vi "Event Receive.vi"(11 "Base Event jettl in":refnum<class "Base Event jettl.lvclass">) -> (2 "Event Msg Strategy":refnum<user-event>, 3 "Base Event jettl out":refnum<class "Base Event jettl.lvclass">)   [LabVIEW 2021, in "jettl.lvlib" / "Base Event jettl.lvlib" / "Base Event jettl.lvclass"]
uses:
  Base Event jettl.lvclass
  Msg Strategy/Msg Strategy/Msg Strategy.lvclass
  Base Event jettl.lvclass/Base Event jettl.ctl
  jettl.lvlib
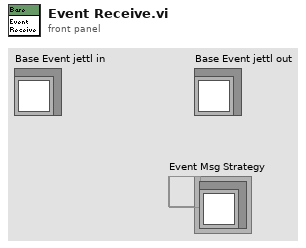
[diagram p1: front panel]
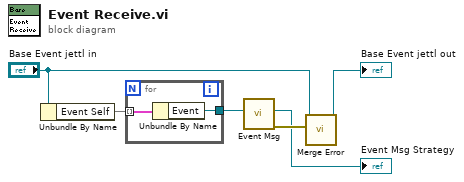
[diagram p0: block diagram]
diagram:
  n1 = Unbundle By Name("Base Event jettl in") -> ("Event Self"=w4:map{string, refnum<data-value>})
  n2 = for {
    tunnel: w4 -> [w8] mode=indexing
    tunnel: [w7] -> w3
    n3 = Unbundle By Name(w8) -> ("Event"=w7:refnum<data-value>)
  }
  n4 = call "Event Msg.vi"("Event"=w3) -> ("error out"=w2:errorcluster, "Event Msg Strategy"=→"Event Msg Strategy":refnum<user-event>)  [unwired: 9 in]
  n5 = call-dynamic "Merge Error.vi"("Error"=w2, "Base Event jettl in"="Base Event jettl in") -> ("Base Event jettl out"=→"Base Event jettl out":refnum<class "Base Event jettl.lvclass">)  [unwired: 9 in]
